vi "Send Email using SMTP Client.vi"(5 "send map":bool, 7 "CC":string="cornelius.krull@mailbox.org", 8 "error in (no error)":errorcluster, 9 "Message":string="Test", 10 "Subject":string="Hallo", 11 "To:":string="cornelius.krull@mailbox.org") -> (0 "error out":errorcluster)   [LabVIEW 2014]
doc: "Uses the SMTP Email Client to send an email to a standard or secure SMTP server."
uses:
  <vilib>/smtpClient/Set Message Text.vi
  <vilib>/smtpClient/LabVIEWSMTPClient.lvlib
panel:
  in  "Sender's Email Address":string="DQN.agent@gmail.com"
  in  "Password":string="holacaracola"
  in  "Enable TLS":bool=TRUE
  in  "Username":string="DQN.agent@gmail.com"
  in  "Port":string="587"
  in  "Outgoing Mail Server (SMTP)":string="smtp.gmail.com"
  # "Overview: Connects to an SMTP Email Server, and sends one or more emails.\nRequirements: LabVIEW Full Development System\nInstructions:\n1. Run the VI.\n2. Configure the Outgoing Mail Server section, then click Configure Server.\n3. Specify the Compose Email content, then click Send Email.\n4. Click Stop to stop the VI."
  # "Outgoing Mail Server"
  # "Compose Email"
  # "Optional Parameters"
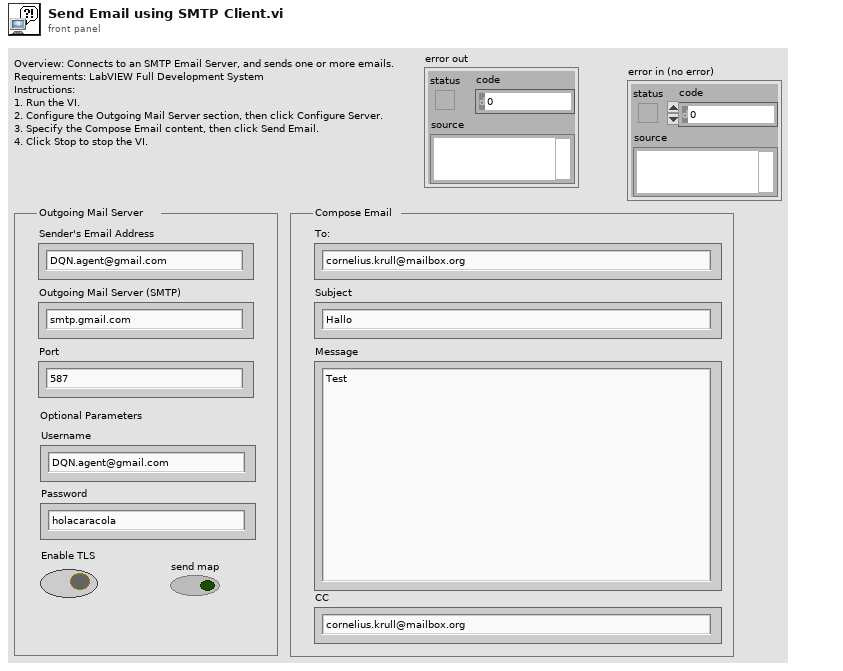
[diagram p1: front panel]
types:
  T1 = typedef "LabVIEWSMTPClient.lvlib/SmtpClientHandle.ctl" = refnum<k1>
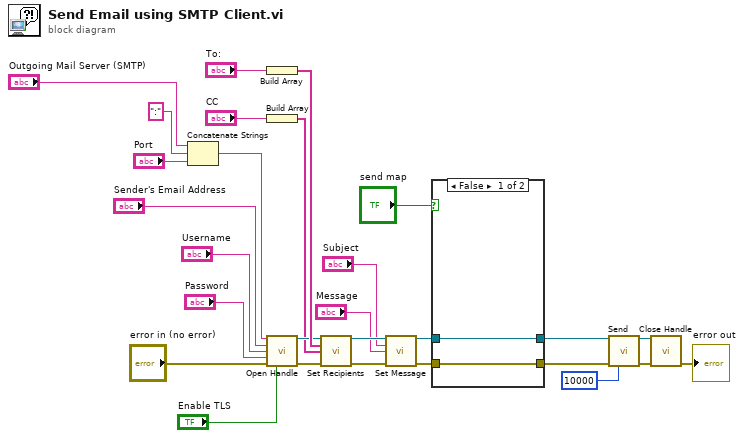
[diagram p0: block diagram]
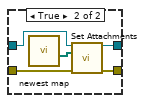
[diagram p2: hidden frame]
diagram:
  n1 = Concatenate Strings("Outgoing Mail Server (SMTP)", ":" ("string"), "Port") -> (w25:string)
  n2 = Build Array("To:") -> (w15:string[])
  n3 = Build Array("CC") -> (w7:string[])
  n4 = call <vilib>:"Open Handle.vi"("server address"=w25, "from"="Sender's Email Address", "username"="Username", "password"="Password", "error in (no error)"="error in (no error)", "use TLS (false)"="Enable TLS") -> ("handle out"=w13:T1, "error out"=w12:errorcluster)  [unwired: 8 in]
  n5 = call <vilib>:"Set Recipients.vi"("handle in"=w13, "to"=w15, "cc"=w7, "error in (no error)"=w12) -> ("handle out"=w19:T1, "error out"=w16:errorcluster)  [unwired: 10 in]
  n6 = call-poly <vilib>:"Set Message.vi"("handle in"=w19, "subject"="Subject", "plain text message"="Message", "error in (no error)"=w16) -> ("handle out"=w5:T1, "error out"=w3:errorcluster)  [unwired: 10 in]
  n7 = case shown="False" "send map" {
    tunnel: w5 -> [w30 w34]
    tunnel: [w30 w33] -> w4
    tunnel: w3 -> [w29 w32]
    tunnel: [w29 w31] -> w2
    frame False {
    }
    frame True {
      n8 = call "newest map.vi"() -> ("newest map"=w35:path[])  [unwired: 11 in]
      n9 = call <vilib>:"Set Attachments.vi"("handle in"=w34, "attachments"=w35, "error in (no error)"=w32) -> ("handle out"=w33:T1, "error out"=w31:errorcluster)  [unwired: 11 in]
    }
  }
  n10 = call <vilib>:"Send.vi"("handle in"=w4, "error in (no error)"=w2, "timeout in ms (10000)"=10000 ("timeout in ms")) -> ("handle out"=w11:T1, "error out"=w10:errorcluster)  [unwired: 10 in, 1 out]
  n11 = call <vilib>:"Close Handle.vi"("handle in"=w11, "error in (no error)"=w10) -> ("error out"=→"error out":errorcluster)  [unwired: 12 in, 1 out]
